vi "Pattern Analysis.vi"() -> ()   [LabVIEW 2013]
uses:
  <vilib>/Analysis/2dsp.llb/Real FFT.vi
  <vilib>/addons/Wavelet Analysis/application.llb/WA Denoise (DWT Real Array).vi
  <vilib>/express/express analysis/Spectral/Block/exnSpectralBlock spectral measurements RMS poly.vi
  <vilib>/express/express analysis/Spectral/Block/exnSpectralBlock spectral measurements RMS WFM.vi
  <vilib>/express/express analysis/Spectral/XNode/ExpressSpectralMeasurementsBlockNode.xnode
  <vilib>/ptbypt/NI_PtbyPt.lvlib
  <vilib>/Analysis/NI_AALPro.lvlib
  <vilib>/addons/_Advanced Signal Processing/NI_AdvSigProcWA.lvlib
panel:
  in  "levels":i32=-1
  in  "wavelet":u16(ring) items=["db02"=0, "db03"=1, "db04"=2, "db05"=3, "db06"=4, "db07"=5, "db08"=6, "db09"=7, "db10"=8, "db11"=9, "db12"=10, "db13"=11, "db14"=12, "Haar"=13, "bior1_3"=14, "bior1_5"=15, "bior2_2"=16, "bior2_4"=17, "bior2_6"=18, "bior2_8"=19, "bior3_1"=20, "bior3_3"=21, "bior3_5"=22, "bior3_7"=23, "bior3_9"=24, "bior4_4 (FBI)"=25, "bior5_5"=38, "bior6_8"=39, "coif1"=26, "coif2"=27, "coif3"=28, "coif4"=29, "coif5"=30, "sym2"=31, "sym3"=32, "sym4"=33, "sym5"=34, "sym6"=35, "sym7"=36, "sym8"=37]
  in  "option for approx coef":u16(ring) items=["None", "Threshold", "Detrend"]
  in  "threshold settings":T1={"thresholding rule"=enum."SURE", "rescaling method"=1, "soft threshold?"=TRUE} {"rescaling method" items=["One", "Single level", "Multiple levels"]}
  out "Intensity Graph":dbl[][](graph)
  out "Fit Data 2":dbl[](graph)
  in  "threshold valley":dbl format="%0.2f"
  in  "threshold peak":dbl format="%0.2f"
  in  "ratio":dbl=0.4 min=0.0 max=1.0
  in  "sample length":i32=100
  out "interpolation value":dbl format="%0.2f"
  in  "polynomial order":i32=2
  out "size(s)":i32
  out "Fit Data":dbl[](graph)
  in  "Index":i32=1136
  out "Selected Pattern Size":i32
  out "WS7 Selected Pattern Data":dbl[](graph)
  out "Pattern Size":i32
  out "Loop Counter":i32
  in  "Stop":bool
  out "WS7 Pattern2 Data":dbl[](graph)
  # "1136"
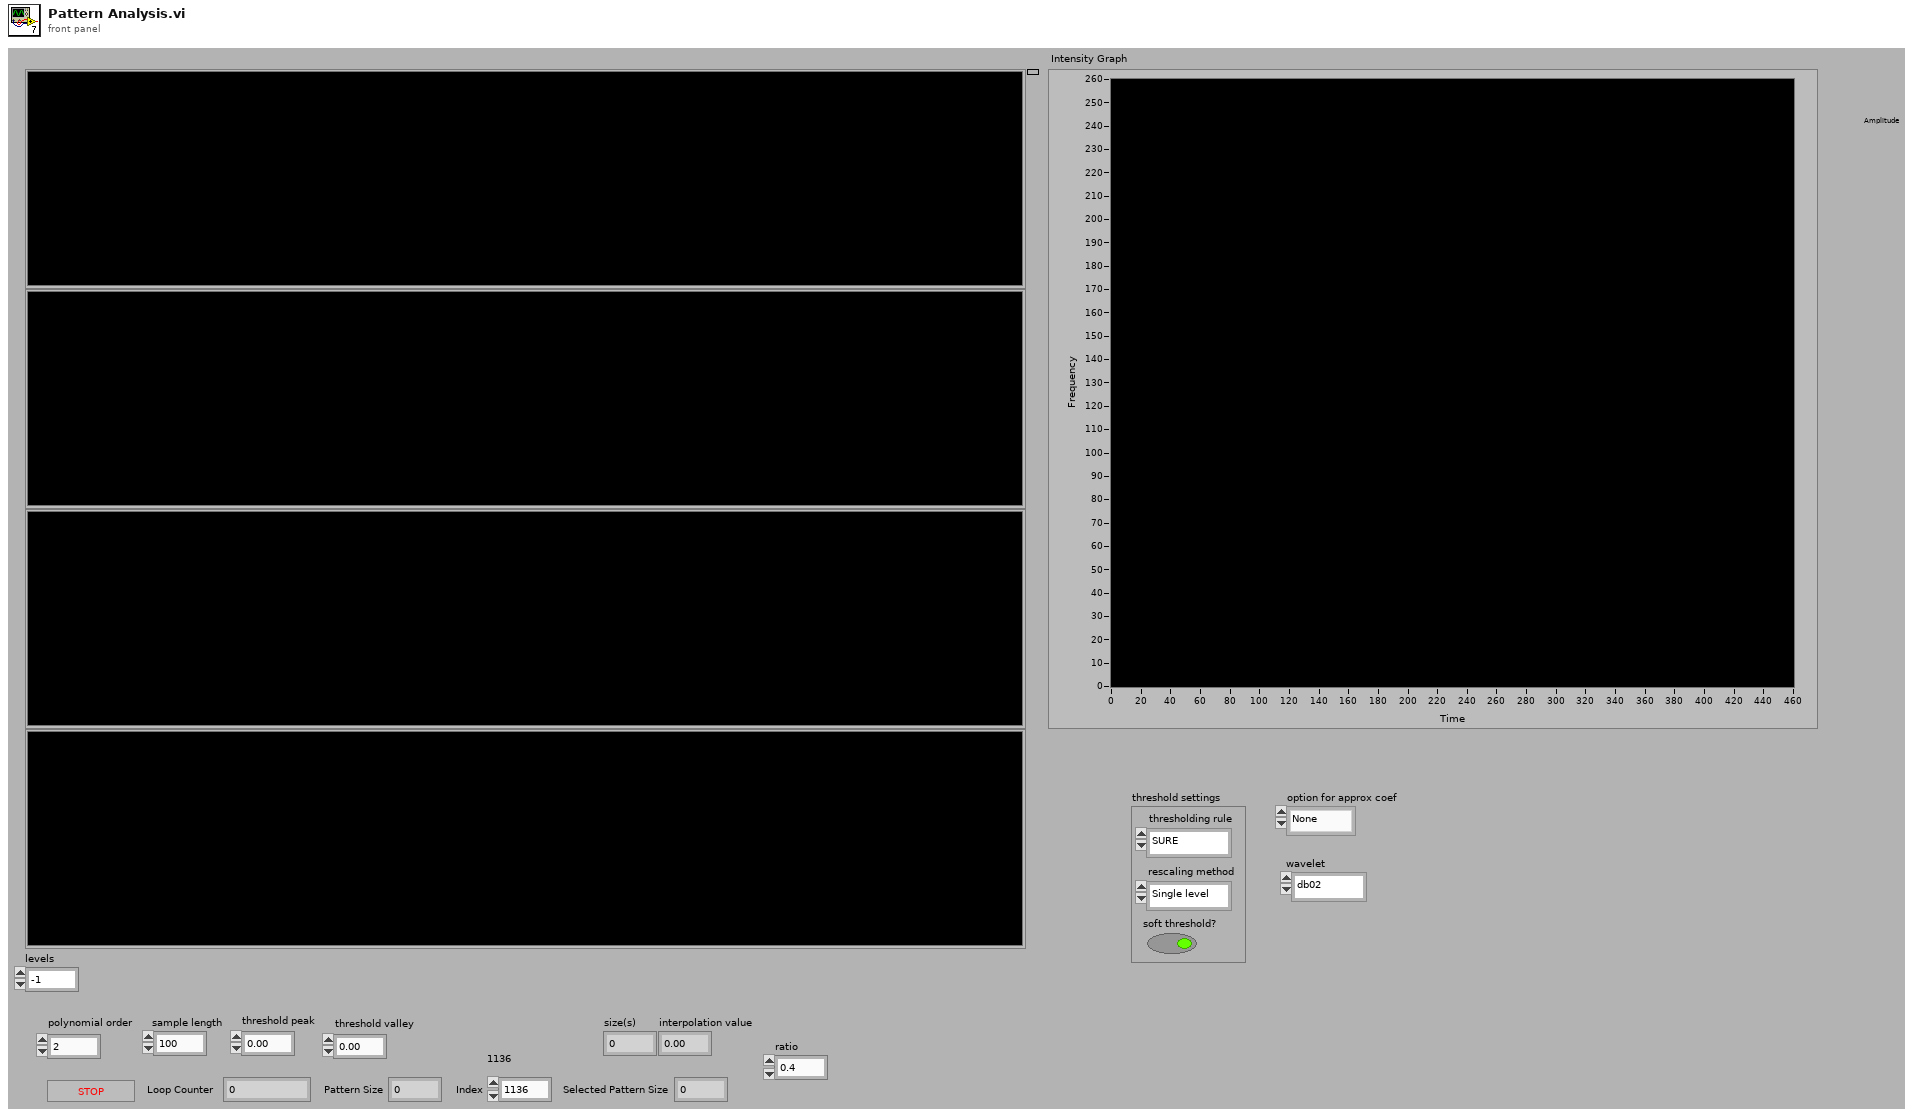
[diagram p1: front panel]
types:
  T1 = cluster{"thresholding rule":enum16{"SURE", "Hybrid", "Universal", "Minimax"}, "rescaling method":u16, "soft threshold?":bool}
  T2 = cluster{"averaging mode":u16, "weighting mode":u16, "number of averages":u32}
  T3 = cluster{"dB On (F)":bool, "unwrap phase (F)":bool, "convert to degree (F)":bool}
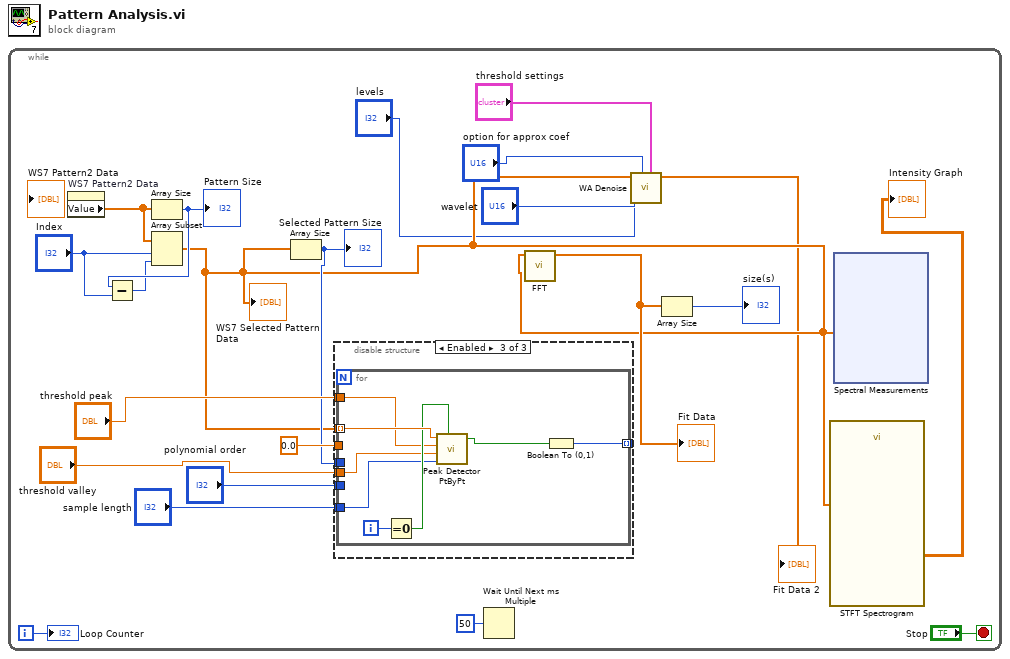
[diagram p0: block diagram]
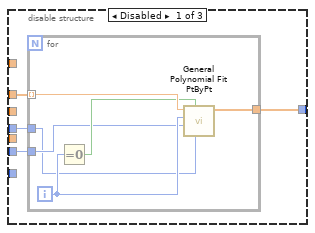
[diagram p2: hidden frame]
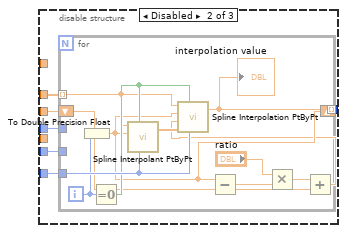
[diagram p3: hidden frame]
diagram:
  n1 = while {
    i -> [w22]
    stop <- "Stop" stop-if-true
    n2 = property on="WS7 Pattern2 Data" class="WFGraph (strict)"() -> ("Value"=w19:dbl[])  [unwired: 2 in, 2 out]
    n3 = Array Size(array=w19) -> (size(s)=w18:i32)
    "Pattern Size" <- w18
    n4 = Subtract(x=w18, y="Index") -> (x-y=w16:i32)
    n5 = Array Subset(array=w19, index="Index", length=w16) -> (w6:dbl[])
    "WS7 Selected Pattern Data" <- w6
    n6 = Array Size(array=w6) -> (size(s)=w8:i32)
    "Selected Pattern Size" <- w8
    n7 = disable-structure shown="Enabled" {
      disable-tunnel: w6 -> [w36 w48 w67]
      disable-tunnel: w8 -> [w35 w47 w66]
      disable-tunnel: [w34 w46 w63] -> _
      disable-tunnel: "polynomial order" -> [w33 w45 w65]
      disable-tunnel: "sample length" -> [_ w44 w64]
      disable-tunnel: 0.0 -> [_ w43 _]
      disable-tunnel: "threshold peak" -> [_ _ w62]
      disable-tunnel: "threshold valley" -> [_ _ w61]
      frame Disabled {
        n8 = for {
          tunnel: w36 -> [w42] mode=indexing
          tunnel: w35 -> [w37]
          tunnel: [w39] -> w34
          tunnel: w33 -> [w38]
          i -> [w41]
          n9 = Equal To 0?(x=w41) -> (x = 0?=w40:bool)
          n10 = call <vilib>:"General Polynomial Fit PtByPt.vi"("sample length"=w37, "initialize"=w40, "polynomial order"=w38, "x"=w41, "y"=w42) -> ("Best Polynomial Fit"=w39:dbl[])  [unwired: 1 in, 3 out]
        }
      }
      frame Disabled {
        n11 = for {
          tunnel: w48 -> [w55] mode=indexing
          tunnel: w47 -> [_]
          tunnel: [w60] -> w46 mode=indexing
          tunnel: w45 -> [_]
          tunnel: w44 -> [w58]
          shift-right: [w50] -> _
          shift-left: w43 -> [w51]
          i -> [w57]
          n12 = To Double Precision Float(number=w57) -> (double precision float=w50:dbl)
          n13 = Equal To 0?(x=w57) -> (x = 0?=w56:bool)
          n14 = call <vilib>:"Spline Interpolant PtByPt.vi"("sample length"=w58, "initialize"=w56, "x"=w50, "y"=w55) -> ("Interpolant"=w59:dbl[])  [unwired: 2 in, 1 out]
          n15 = Subtract(x=w50, y=w51) -> (x-y=w52:dbl)
          n16 = Multiply(x="ratio", y=w52) -> (x*y=w53:dbl)
          n17 = Add(x=w53, y=w51) -> (x+y=w49:dbl)
          n18 = call <vilib>:"Spline Interpolation PtByPt.vi"("sample length"=w58, "initialize"=w56, "Interpolant"=w59, "x value"=w49, "x"=w50, "y"=w55) -> ("interpolation value"=w60:dbl)  [unwired: 1 out]
          "interpolation value" <- w60
        }
      }
      frame Enabled {
        n19 = for {
          tunnel: w67 -> [w74] mode=indexing
          tunnel: w66 -> [_]
          tunnel: w65 -> [_]
          tunnel: w64 -> [w70]
          tunnel: [w71] -> w63 mode=indexing
          tunnel: w62 -> [w69]
          tunnel: w61 -> [w68]
          i -> [w75]
          n20 = Equal To 0?(x=w75) -> (x = 0?=w73:bool)
          n21 = call <vilib>:"Peak Detector PtByPt.vi"("x"=w74, "threshold peak"=w69, "threshold valley"=w68, "width"=w70, "initialize"=w73) -> ("peak"=w72:bool)  [unwired: 2 out]
          n22 = Boolean To (0,1)(Boolean=w72) -> (0, 1=w71:i16)
        }
      }
    }
    n23 = Wait Until Next ms Multiple(millisecond multiple=u32 50) -> ()  [unwired: 1 out]
    n24 = call-poly <vilib>:"FFT.vi"("X"=w6) -> ("FFT {X}"=w9:cdb[])  [unwired: 9 in, 1 out]
    "Fit Data" <- w9
    n25 = call-poly <vilib>:"WA Denoise.vi"("threshold settings"="threshold settings", "option for approx coef"="option for approx coef", "wavelet"="wavelet", "levels"="levels", "signal"=w6) -> ("denoised signal"=→"Fit Data 2":dbl[])  [unwired: 5 in, 1 out]
    n26 = Array Size(array=w9) -> (size(s)=→"size(s)":i32)
    n27 = call "STFT Spectrogram"("Signal"=w6) -> ("Spectrogram"=→"Intensity Graph":dbl[][])  [unwired: 6 in, 4 out]
    n28 = xnode "Spectral Measurements"("Signals"=w6) -> ()  [unwired: 1 in, 3 out]
    "Loop Counter" <- w22
  }
